vi "Secure WebSocket Server Test.vi"() -> ()   [LabVIEW 2013]
uses:
  NI OpenSSL Socket/SSL_Lib/SSL-Lib/Library Paths.ctl
  NI OpenSSL Socket/SSL Server Context/SSL Server Context.lvclass/SSL Server Context.ctl
  NI OpenSSL Socket/SSL Server Context/SSL Server Context.lvclass
  NI OpenSSL Socket/SSL Server Socket/SSL Server Socket.lvclass
  <vilib>/MediaMongrels Ltd/WebSockets/WebSockets/WebSocket Server/WebSocket Server.lvclass
  <vilib>/MediaMongrels Ltd/WebSockets/WebSockets/WebSocket/WebSocket.lvclass/WebSocket.ctl
  NI OpenSSL Socket/SSL Server Context/Write Certificate Chain File.vi
  NI OpenSSL Socket/SSL Server Context/Write Private Key.vi
  <vilib>/MediaMongrels Ltd/WebSockets/WebSockets/WebSocket/Read Return Headers.vi
  NI OpenSSL Socket/SSL_Lib/SSL-Lib/SSL-Lib.lvclass
panel:
  out "Sent Data":string
  out "error out":errorcluster
  in  "Stop":bool
  out "RX Data":string
  out "Return Headers":variant
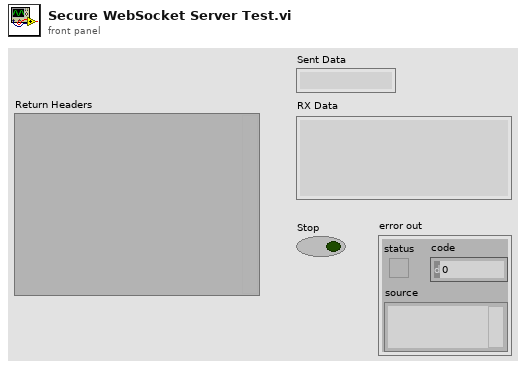
[diagram p1: front panel]
types:
  T1 = typedef "OpenSSL Socket.lvlib/SSL-Lib.lvclass/Library Paths.ctl" = cluster{"SSL Library Path":path, "Crypto Library Path":path}
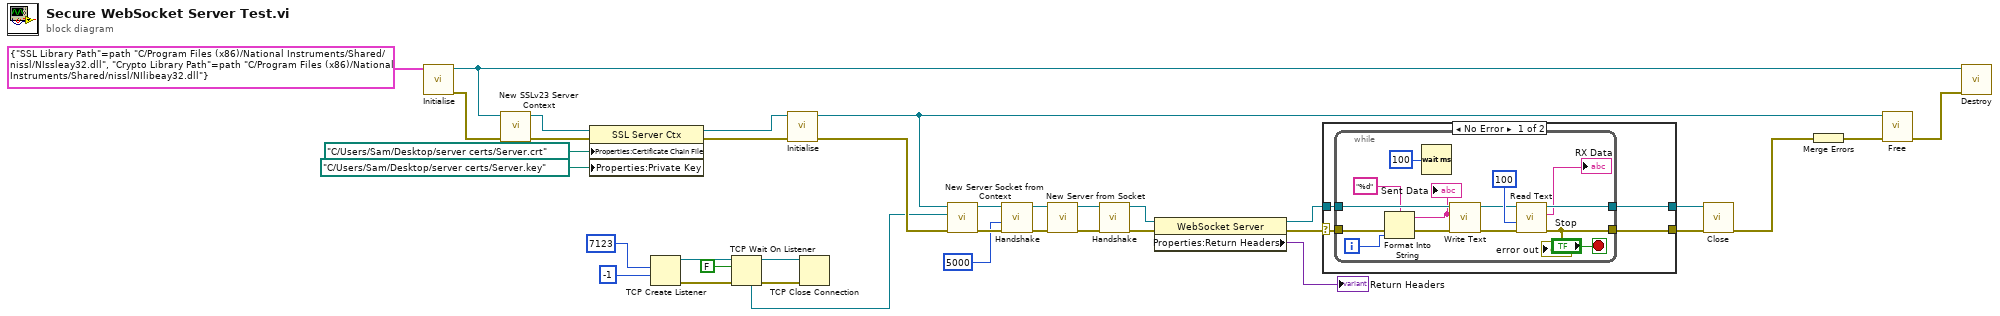
[diagram p0: block diagram]
diagram:
  n1 = call "Initialise.vi"("Library Paths"=T1 {"SSL Library Path"=path "C:/Program Files (x86)/National Instruments/Shared/nissl/NIssleay32.dll", "Crypto Library Path"=path "C:/Program Files (x86)/National Instruments/Shared/nissl/NIlibeay32.dll"}) -> ("error out"=w27:errorcluster, "SSL-Lib out"=w25:refnum<class "SSL-Lib.lvclass">)  [unwired: 9 in]
  n2 = call "New SSLv23 Server Context.vi"("error in (no error)"=w27, "SSL-Lib"=w25) -> ("error out"=w26:errorcluster, "SSL Client Context out"=w21:refnum<class "SSL Server Context.lvclass">)  [unwired: 8 in]
  n3 = property class="SSL Server Ctx"(reference=w21, error in=w26, "Properties:Certificate Chain File"=path "C:/Users/Sam/Desktop/server certs/Server.crt", "Properties:Private Key"=path "C:/Users/Sam/Desktop/server certs/Server.key") -> (reference out=w20:refnum<class "SSL Server Context.lvclass">, error out=w22:errorcluster)
  n4 = TCP Create Listener(9:-1 ("timeout ms (25000)"), 10:u16 7123 ("port")) -> (0:w8:errorcluster, 3:w11:refnum<k5>)  [unwired: 3 in, 1 out]
  n5 = TCP Wait On Listener(8:w8, 10:FALSE ("resolve remote address (T)"), 11:w11) -> (0:w10:errorcluster, 3:w9:refnum<k5>, 4:w2:refnum<k5>)  [unwired: 1 in, 2 out]
  n6 = call-dynamic "Initialise.vi"("error in (no error)"=w22, "OpenSSL Server Context in"=w20) -> ("error out"=w18:errorcluster, "OpenSSL Server Context out"=w19:refnum<class "SSL Server Context.lvclass">)  [unwired: 8 in]
  n7 = TCP Close Connection(connection ID=w9, error in (no error)=w10) -> ()  [unwired: 1 in, 2 out]
  n8 = call "New Server Socket from Context.vi"("error in (no error)"=w18, "TCP Refnum"=w2, "SSL Server Ctx"=w19) -> ("error out"=w6:errorcluster, "SSL Server Skt out"=w7:refnum<class "SSL Server Socket.lvclass">)  [unwired: 7 in]
  n9 = call-dynamic "Handshake.vi"("error in (no error)"=w6, "Timeout (5000ms)"=u32 5000, "OpenSSL in"=w7) -> ("error out"=w5:errorcluster, "OpenSSL out"=w4:refnum<class "SSL Server Socket.lvclass">)  [unwired: 7 in]
  n10 = call <vilib>:"New Server from Socket.vi"("error in (no error)"=w5, "Socket"=w4) -> ("error out"=w36:errorcluster, "WebSocket Server out"=w35:refnum<class "WebSocket Server.lvclass">)  [unwired: 8 in]
  n11 = call-dynamic "Handshake.vi"("error in (no error)"=w36, "WebSocket Connection in"=w35) -> ("error out"=w34:errorcluster, "WebSocket Connection out"=w33:refnum<class "WebSocket Server.lvclass">)  [unwired: 8 in]
  n12 = property class="WebSocket Server"(reference=w33, error in=w34) -> (reference out=w31:refnum<class "WebSocket Server.lvclass">, error out=w1:errorcluster, "Properties:Return Headers"=→"Return Headers":variant)
  n13 = case shown="No Error" w1 {
    selector: w1 -> [w37 w54]
    tunnel: w31 -> [w40 w55]
    tunnel: [w39 w54] -> w30
    tunnel: [w38 w55] -> w29
    frame No Error {
      n14 = while {
        tunnel: w37 -> [w45]
        tunnel: w40 -> [w48]
        tunnel: [w53] -> w39
        tunnel: [w52] -> w38
        i -> [w43]
        stop <- "Stop" stop-if-true
        n15 = Format Into String(format string="%d", w43) -> (resulting string=w44:string)  [unwired: 2 in, 1 out]
        "Sent Data" <- w44
        n16 = Wait (ms)(milliseconds to wait=u32 100) -> ()  [unwired: 1 out]
        n17 = call-dynamic "Write Text.vi"("error in (no error)"=w45, "String Data"=w44, "WebSocket in"=w48) -> ("error out"=w46:errorcluster, "WebSocket out"=w47:refnum<class "WebSocket Server.lvclass">)  [unwired: 7 in]
        n18 = call-dynamic "Read Text.vi"("error in (no error)"=w46, "timeout ms (5000)"=100, "WebSocket in"=w47) -> ("error out"=w53:errorcluster, "Data"=→"RX Data":string, "WebSocket out"=w52:refnum<class "WebSocket Server.lvclass">)  [unwired: 6 in]
        "error out" <- w53
      }
    }
    frame Error {
    }
  }
  n19 = call-dynamic "Close.vi"("error in (no error)"=w30, "WebSocket in"=w29) -> ("error out"=w23:errorcluster)  [unwired: 9 in]
  n20 = Merge Errors(w23) -> (w17:errorcluster)
  n21 = call-dynamic "Free.vi"("error in (no error)"=w17, "OpenSSL Context in"=w19) -> ("error out"=w24:errorcluster)  [unwired: 9 in]
  n22 = call "Destroy.vi"("error in (no error)"=w24, "SSL-Lib in"=w25) -> ()  [unwired: 9 in, 1 out]
